vi "Calculate Vertex Array.vi"(8 "error in (no error)":errorcluster, 10 "2D Compass Datatype.lvclass in":refnum<class "2D Compass Datatype.lvclass">, 11 "Plot Representation In":T1) -> (0 "error out":errorcluster, 2 "2D Compass Datatype.lvclass out":refnum<class "2D Compass Datatype.lvclass">, 3 "Plot Representation Out":T1)   [LabVIEW 2017, in "2D Compass Datatype.lvclass"]
uses:
  <vilib>/Math Plots/2D Math Plots/2D Compass/2D Compass Datatype/2D Compass Datatype.lvclass
  <vilib>/Math Plots/2D Math Plots/2D Plot/2D Plot/Typedef/Plot Representation.ctl
  <vilib>/Math Plots/2D Math Plots/2D Plot/2D Plot/Typedef/Range Cluster.ctl
  <vilib>/Math Plots/2D Math Plots/2D Compass/2D Compass Datatype/2D Compass Datatype.lvclass/2D Compass Datatype.ctl
  <vilib>/Math Plots/2D Math Plots/2D Plot/2D Plot/2D Plot.lvclass
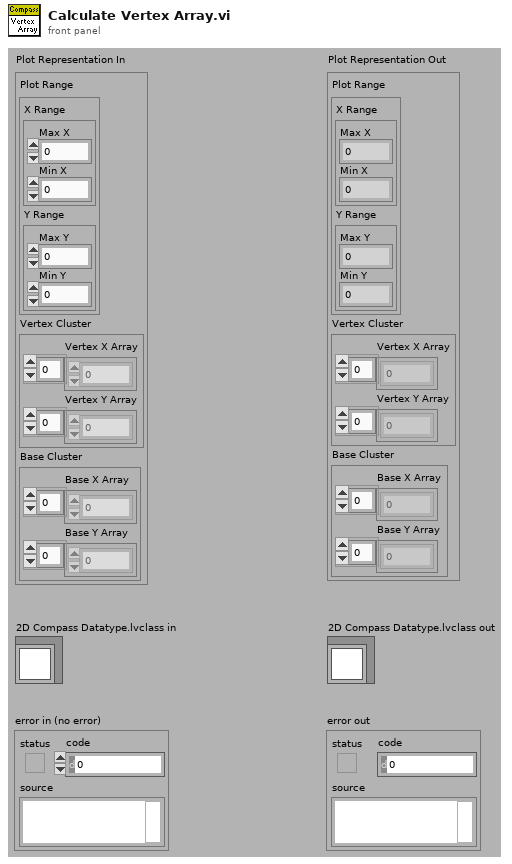
[diagram p1: front panel]
types:
  T1 = typedef "2D Plot.lvclass/Plot Representation.ctl" = cluster{"Plot Range":T2, "Vertex Cluster":cluster{"Vertex X Array":dbl[], "Vertex Y Array":dbl[]}, "Base Cluster":cluster{"Base X Array":dbl[], "Base Y Array":dbl[]}}
  T2 = typedef "2D Plot.lvclass/Range Cluster.ctl" = cluster{"X Range":cluster{"Max X":dbl, "Min X":dbl}, "Y Range":cluster{"Max Y":dbl, "Min Y":dbl}}
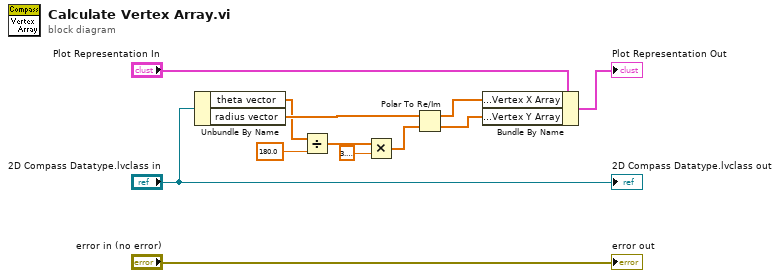
[diagram p0: block diagram]
diagram:
  n1 = Unbundle By Name("2D Compass Datatype.lvclass in") -> ("theta vector"=w7:dbl[], "radius vector"=w8:dbl[])
  n2 = Divide(x=w7, y=180.0) -> (x/y=w5:dbl[])
  n3 = Multiply(x=w5, y=3.141592653589793) -> (x*y=w6:dbl[])
  n4 = Polar To Re/Im(2:w6, 3:w8) -> (0:w1:dbl[], 1:w2:dbl[])
  n5 = Bundle By Name(cluster="Plot Representation In", "Vertex Cluster.Vertex X Array"=w2, "Vertex Cluster.Vertex Y Array"=w1) -> (→"Plot Representation Out":T1)
  "2D Compass Datatype.lvclass out" <- "2D Compass Datatype.lvclass in"
  "error out" <- "error in (no error)"
